vi "AreaEnclosed.vi"(10 "H":dbl[](array[numeric]), 11 "B":dbl[](array[numeric])) -> (3 "Area":dbl)   [LabVIEW 2019]
panel:
  out "output array":dbl[](array[numeric])
  out "AreaArray":dbl[](array[numeric])
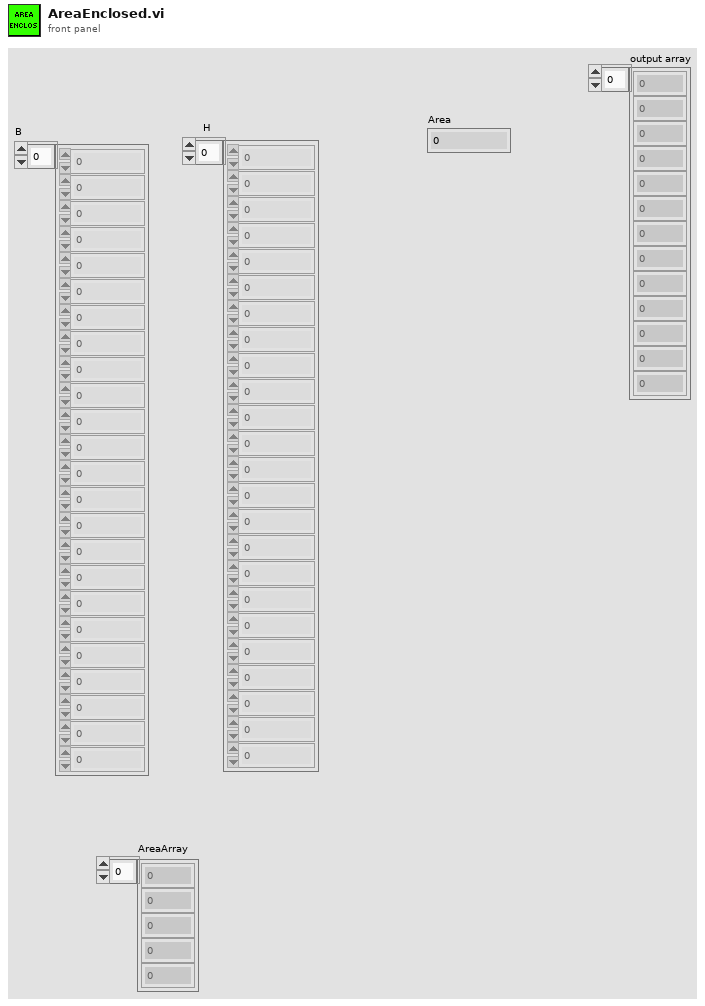
[diagram p1: front panel]
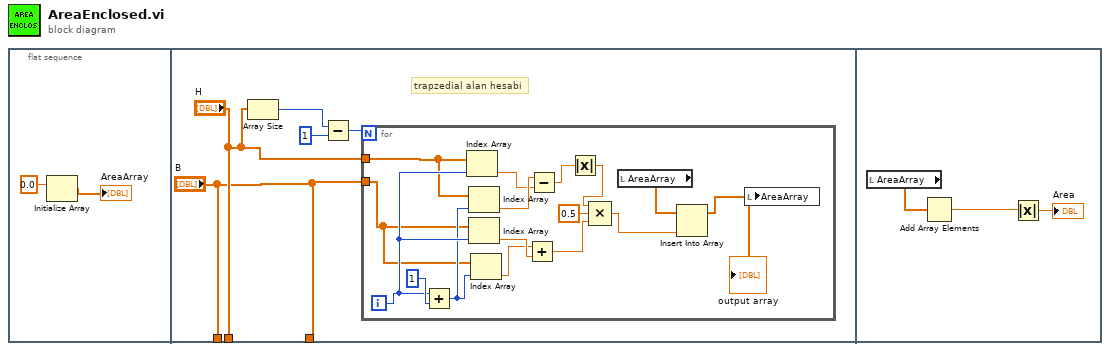
[diagram p0: block diagram]
diagram:
  n1 = flat-sequence {
    tunnel: ["H"] -> _
    tunnel: ["B"] -> _
    tunnel: ["B"] -> _
    frame #0 {
      n2 = Initialize Array(0.0 ("element")) -> (→"AreaArray":dbl[])  [unwired: 1 in]
    }
    frame #1 {
      # "trapzedial alan hesabi"
      n3 = Array Size(array="H") -> (size(s)=w6:i32)
      n4 = Subtract(x=w6, y=1) -> (x-y=w7:i32)
      n5 = for {
        N: w7 -> [_]
        tunnel: "H" -> [w21]
        tunnel: "B" -> [w19]
        i -> [w22]
        n6 = Add(x=w22, y=1) -> (x+y=w20:i32)
        n7 = Index Array(array=w21, index=w22) -> (element=w17:dbl)
        n8 = Index Array(array=w21, index=w20) -> (element=w18:dbl)
        n9 = Index Array(array=w19, index=w22) -> (element=w16:dbl)
        n10 = Index Array(array=w19, index=w20) -> (element=w15:dbl)
        n11 = Add(x=w15, y=w16) -> (x+y=w14:dbl)
        n12 = Subtract(x=w18, y=w17) -> (x-y=w9:dbl)
        n13 = Absolute Value(x=w9) -> (abs(x)=w8:dbl)
        n14 = Compound Arithmetic op=MULTIPLY(w8, 0.5 ("value"), w14) -> (w10:dbl)
        n15 = local read "AreaArray"() -> (w12:dbl[])
        n16 = Insert Into Array(array=w12, new element=w10) -> (w11:dbl[])  [unwired: 1 in]
        "output array" <- w11
        n17 = local write "AreaArray"(w11) -> ()
      }
    }
    frame #2 {
      n18 = local read "AreaArray"() -> (w26:dbl[])
      n19 = Add Array Elements(numeric array=w26) -> (sum=w25:dbl)
      n20 = Absolute Value(x=w25) -> (abs(x)=→"Area":dbl)
    }
  }
